vi "Execute LShftReg Handle.vi"(4 "Menu Item Tag Suffix":string, 8 "错误输入（无错误）":errorcluster, 11 "左侧移位寄存器输入":refnum<vi>) -> (0 "错误输出":errorcluster)   [LabVIEW 2020]
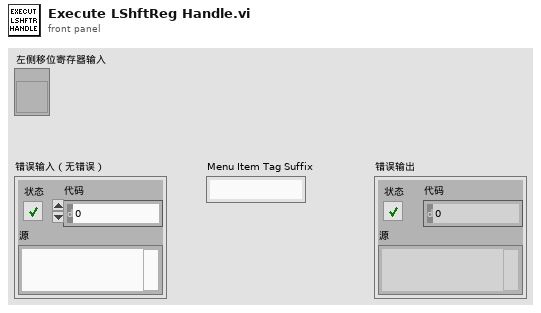
[diagram p1: front panel]
types:
  T1 = typedef "LVRectTypeDef.ctl" = cluster{"Left":i16, "Top":i16, "Right":i16, "Bottom":i16}
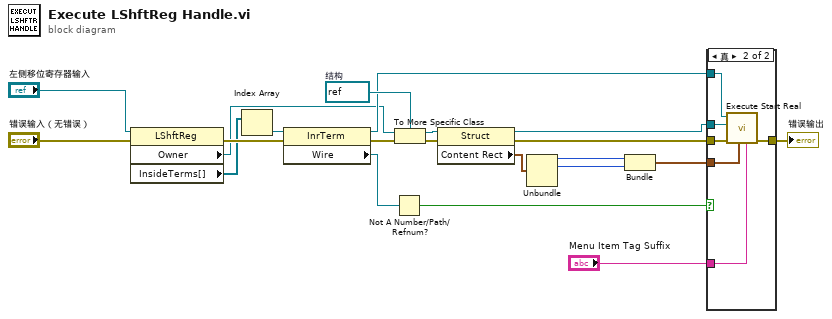
[diagram p0: block diagram]
diagram:
  w11 = refnum<vi> refnum  # 结构
  n1 = property class="LShftReg"(reference="左侧移位寄存器输入", error in="错误输入（无错误）") -> (error out=w20:errorcluster, "Owner"=w1:refnum<vi>, "InsideTerms[]"=w5:refnum<vi>[])  [unwired: 1 out]
  n2 = Index Array(array=w5) -> (element=w6:refnum<vi>)  [unwired: 1 in]
  n3 = property class="InrTerm"(reference=w6, error in=w20) -> (reference out=w8:refnum<vi>, error out=w19:errorcluster, "Wire"=w2:refnum<vi>)
  n4 = Not A Number/Path/Refnum?(number/path/refnum=w2) -> (NaN/Path/Refnum?=w9:bool)
  n5 = To More Specific Class(target class=w11, reference=w1, error in=w19) -> (specific class reference=w13:refnum<vi>, error out=w10:errorcluster)
  n6 = property class="Struct"(reference=w13, error in=w10) -> (reference out=w14:refnum<vi>, error out=w12:errorcluster, "Content Rect"=w15:T1)
  n7 = Unbundle(w15) -> ("Left"=w16:i16, "Top"=w17:i16)  [unwired: 2 out]
  n8 = Bundle("Left"=w16, "Top"=w17) -> (w18:cluster{"Left":i16, "Top":i16})  [unwired: 1 in]
  n9 = case shown="真" w9 {
    tunnel: w12 -> [w22 w28]
    tunnel: w14 -> [_ w27]
    tunnel: "Menu Item Tag Suffix" -> [_ w25]
    tunnel: w8 -> [_ w26]
    tunnel: w18 -> [_ w24]
    tunnel: [w22 w23] -> w21
    frame False {
    }
    frame True {
      n10 = call "Execute Start Real.vi"("Menu Item Tag Suffix"=w25, "相对位置原点"=w24, "错误输入（无错误）"=w28, "所有者引用句柄"=w27, "接线端输入"=w26) -> ("错误输出"=w23:errorcluster)  [unwired: 6 in]
    }
  }
  "错误输出" <- w21
